vi "PhotonCamera_SetPipelineIndex.vi"(9 "PipelineIndex":i32, 11 "CameraName":string) -> ()   [LabVIEW 2019, in "PhotonVisionLib.lvlib"]
doc: "Allows the user to select the active pipeline index.\n \nInputs:\n - cameraName -- The nickname of the camera (found in the PhotonVision UI).\n - index The active pipeline index.\n\nOutputs:\n - >none<"
uses:
  PhotonVisionLib.lvlib
  <vilib>/Rock Robotics/Network Tables/NT Write Number.vi
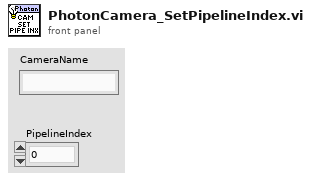
[diagram p1: front panel]
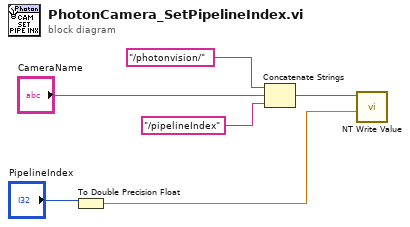
[diagram p0: block diagram]
diagram:
  n1 = To Double Precision Float(number="PipelineIndex") -> (double precision float=w1:dbl)
  n2 = Concatenate Strings("/photonvision/", "CameraName", "/pipelineIndex") -> (w3:string)
  n3 = call-poly <vilib>:"NT Write Value.vi"("Numeric"=w1, "Name"=w3) -> ()  [unwired: 9 in, 1 out]
